vi "SVA 4MV6 P04 CCE RRMA .vi"() -> ()   [LabVIEW 2020]
doc: "Ceballos Conde Emanuel Rodríguez Ramírez Miguel Ángel 4MV6 Sistemas de visión artificial 2022/1\nEste vi devuelve el nombre y firma de una imagen de entrada en formato bmg utilizando la correlacion cruzada con las firmas de distintas figuras guardadas en memoria"
uses:
  SVA 4MV6 P04 CCE RRMA.ctl
  <vilib>/Analysis/2dsp.llb/1D Auto Correlation (DBL).vi
  <vilib>/Analysis/2dsp.llb/1D Cross Correlation (DBL).vi
  <vilib>/Analysis/NI_AALPro.lvlib
panel:
  out "Figura detectada":string
  out "Firma de la imagen":dbl[](graph)
  in  "iniciar":bool
  in  "stop":bool
  out "imagen":picture
  in  "Path":path
  # "Ceballos Conde Emanuel\nRodríguez Ramírez Miguel Ángel\n4MV6\nSistemas de visión artificial\n2022/1"
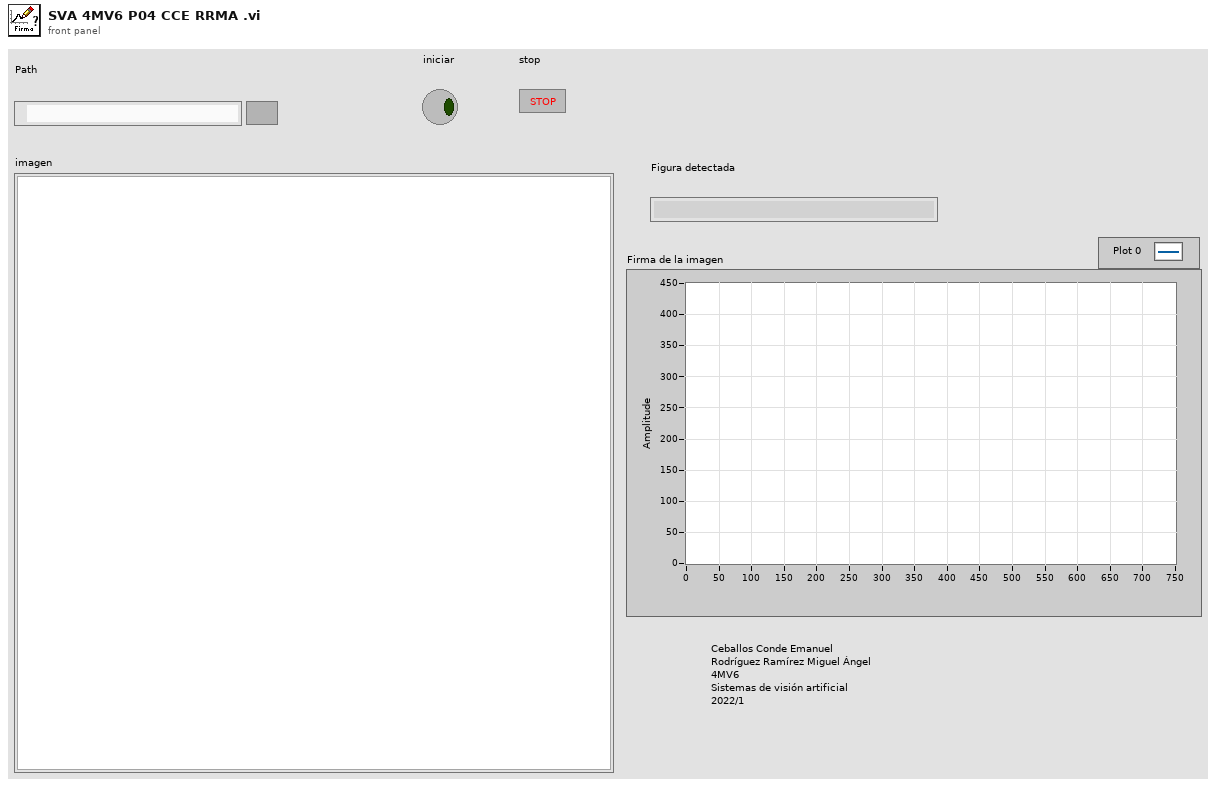
[diagram p1: front panel]
types:
  T1 = typedef "SVA 4MV6 P04 CCE RRMA.ctl" = enum16{"espera", "firma"}
  T2 = typedef "imagedata.ctl" = cluster{"image type":i32, "image depth":i32, "image":u8[], "mask":u8[], "colors":u32[], "Rectangle":cluster{"left":i16, "top":i16, "right":i16, "bottom":i16}}
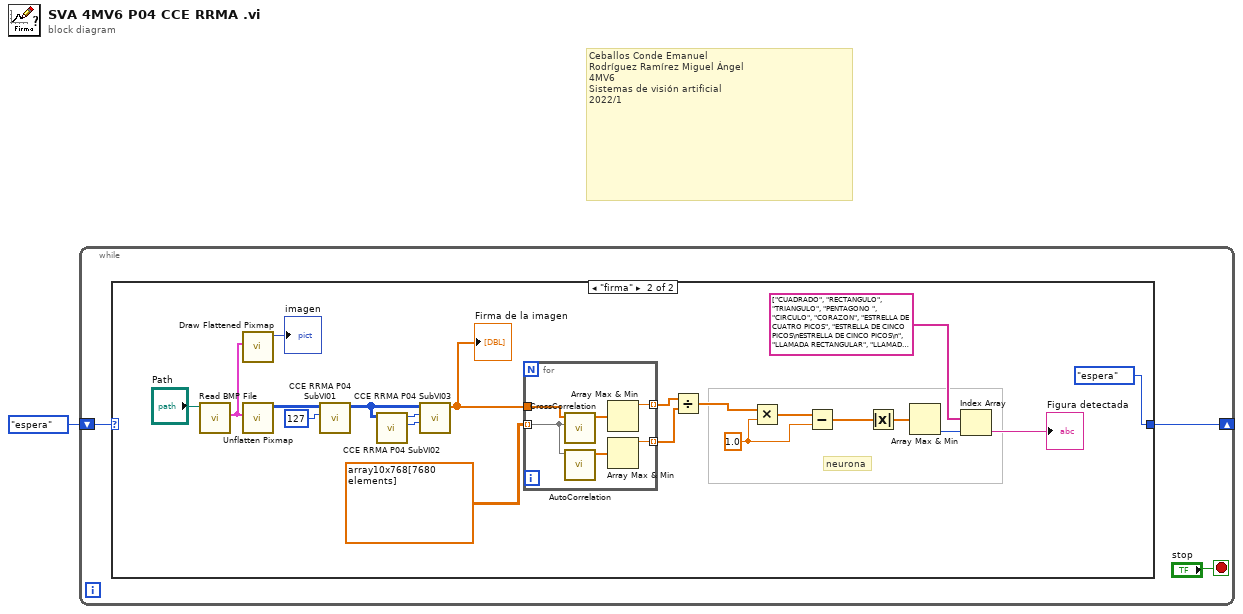
[diagram p0: block diagram]
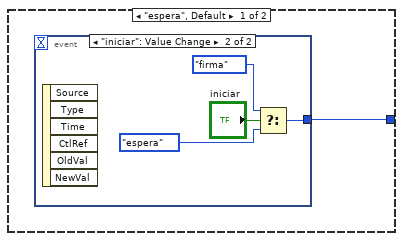
[diagram p2: hidden frame]
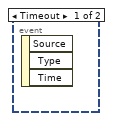
[diagram p3: hidden frame]
diagram:
  # "Ceballos Conde Emanuel\nRodríguez Ramírez Miguel Ángel\n4MV6\nSistemas de visión artificial\n2022/1"
  n1 = while {
    shift-right: [w2] -> _
    shift-left: SVA_4MV6_P04_CCE_RRMA."espera" -> [w4]
    stop <- "stop" stop-if-true
    n2 = case shown="\"firma\"" w4 {
      tunnel: [w5 SVA_4MV6_P04_CCE_RRMA."espera"] -> w2
      frame "espera", Default {
        n3 = event shown="[1] \"iniciar\": Value Change" {
          selector: _ -> [_ _]
          dyn-events: _ -> [_ _]
          timeout: _ -> [_ _]
          tunnel: [_ w6] -> w5
          event Timeout {
            n4 = event-data() -> ()  [unwired: 1 in, 3 out]
          }
          event "iniciar": Value Change {
            n5 = event-data() -> ()  [unwired: 1 in, 6 out]
            n6 = Select(t=SVA_4MV6_P04_CCE_RRMA."firma", s="iniciar", f=SVA_4MV6_P04_CCE_RRMA."espera") -> (s? t:f=w6:T1)
          }
        }
      }
      frame "firma" {
        w18 = 1.0
        # "neurona"
        n7 = call <vilib>:"Read BMP File.vi"("path to BMP file"="Path") -> ("image data"=w28:T2)  [unwired: 8 in, 2 out]
        n8 = call <vilib>:"Draw Flattened Pixmap.vi"("image data"=w28) -> ("new picture"=→"imagen":picture)  [unwired: 8 in]
        n9 = call <vilib>:"Unflatten Pixmap.vi"("image data"=w28) -> ("24-bit pixmap"=w25:u32[][])  [unwired: 4 in, 6 out]
        n10 = call "CCE RRMA P04 SubVI01.vi"("24-bit pixmap"=w25, "umbral superior"=u32 127 ("umbral")) -> ("Array"=w24:u32[][])  [unwired: 8 in]
        n11 = call "CCE RRMA P04 SubVI02.vi"("Array"=w24) -> ("cy"=w22:u32, "cx"=w23:u32)  [unwired: 9 in]
        n12 = call "CCE RRMA P04 SubVI03.vi"("Cy"=w22, "Cx"=w23, "imagen"=w24) -> ("firma"=w10:dbl[])  [unwired: 8 in]
        "Firma de la imagen" <- w10
        n13 = for {
          tunnel: w10 -> [w36]
          tunnel: dbl[][] array10x768[7680 elements] ("firma") -> [w34] mode=indexing
          tunnel: [w33] -> w21 mode=indexing
          tunnel: [w32] -> w13 mode=indexing
          n14 = call-poly <vilib>:"CrossCorrelation.vi"("Y"=w34, "X"=w36) -> ("Rxy"=w31:dbl[])  [unwired: 8 in, 1 out]
          n15 = call-poly <vilib>:"AutoCorrelation.vi"("X"=w34) -> ("Rxx"=w35:dbl[])  [unwired: 9 in, 1 out]
          n16 = Array Max & Min(array=w31) -> (max value=w32:dbl)  [unwired: 3 out]
          n17 = Array Max & Min(array=w35) -> (max value=w33:dbl)  [unwired: 3 out]
        }
        n18 = Divide(x=w13, y=w21) -> (x/y=w20:dbl[])
        n19 = Multiply(x=w20, y=w18) -> (x*y=w19:dbl[])
        n20 = Subtract(x=w19, y=w18) -> (x-y=w17:dbl[])
        n21 = Absolute Value(x=w17) -> (abs(x)=w15:dbl[])
        n22 = Array Max & Min(array=w15) -> (min index (indices)=w14:i32)  [unwired: 3 out]
        n23 = Index Array(array=string[] ["CUADRADO", "RECTANGULO", "TRIANGULO", "PENTAGONO ", "CIRCULO", "CORAZON", "ESTRELLA DE CUATRO PICOS", "ESTRELLA DE CINCO PICOS\nESTRELLA DE CINCO PICOS\n", "LLAMADA RECTANGULAR", "LLAMADA DE ELIPSE"], index=w14) -> (element=→"Figura detectada":string)
      }
    }
  }
